vi "Autonomous.vi"   [LabVIEW 2019]
doc: "This VI starts when autonomous period begins, and will automatically be terminated when it ends. You can carry out timed or sensor driven operations directly to I/O or to subsystems without needing to return to the caller."
uses:
  <vilib>/Rock Robotics/WPI/Utilities/WPI_GetSetVariantRefNum.vi
  <vilib>/Rock Robotics/Network Tables/NT Read String.vi
types:
  T1 = typedef "WPI_JoystickDevRef.ctl" = cluster{"Device":T2}
  T2 = typedef "WPI_JoystickDeviceEnum.ctl" = enum16{"USB 0", "USB 1", "USB 2", "USB 3", "USB 4", "USB 5"}
  T3 = typedef "Command Status Info.ctl" = cluster{"Name":string, "Status":T4, "notifier out":T5}
  T4 = typedef "Completion Status.ctl" = enum16{"Successful", "Aborted", "Incomplete"}
  T5 = typedef "Completion Notifier.ctl" = refnum<notifier>
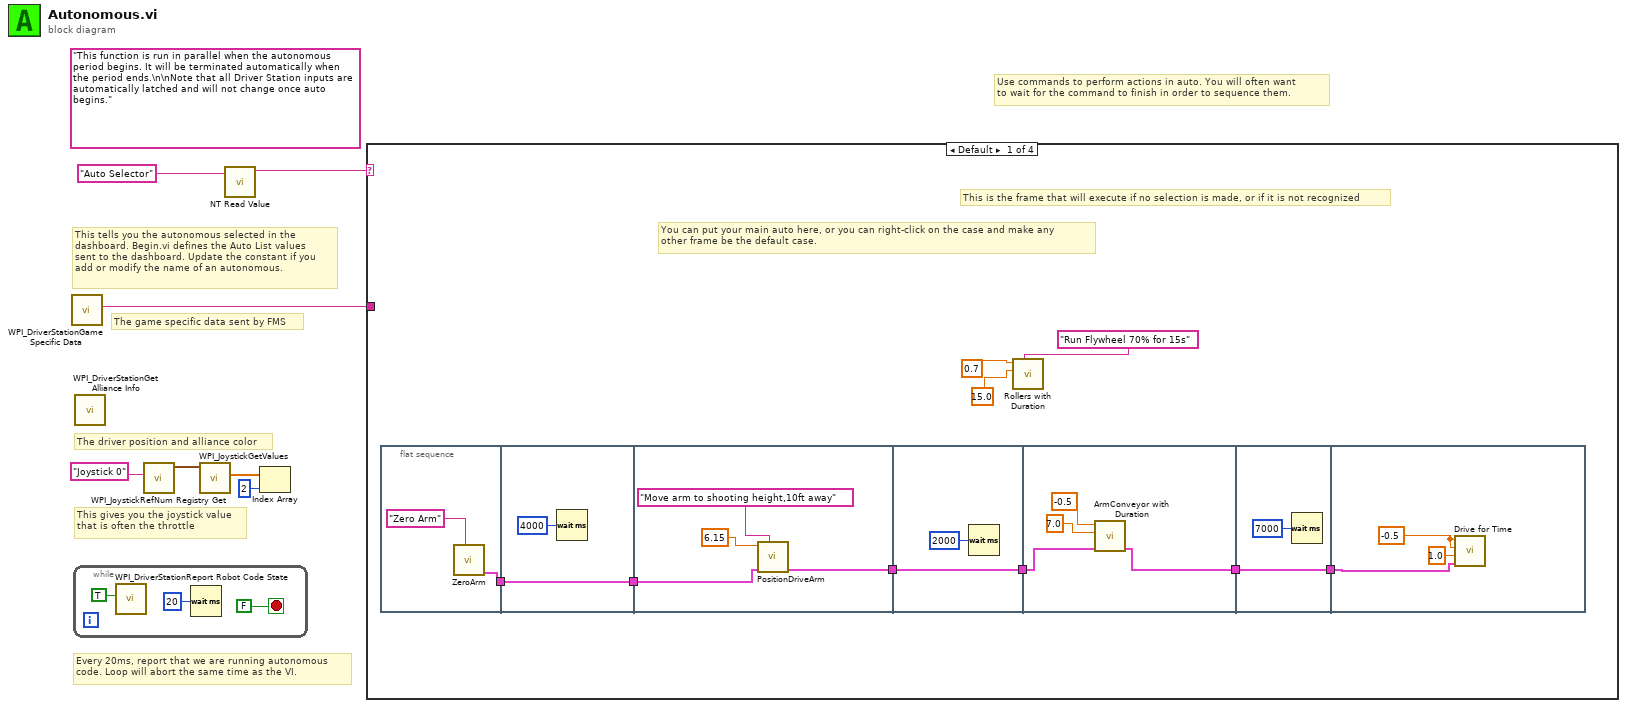
[diagram p0: block diagram]
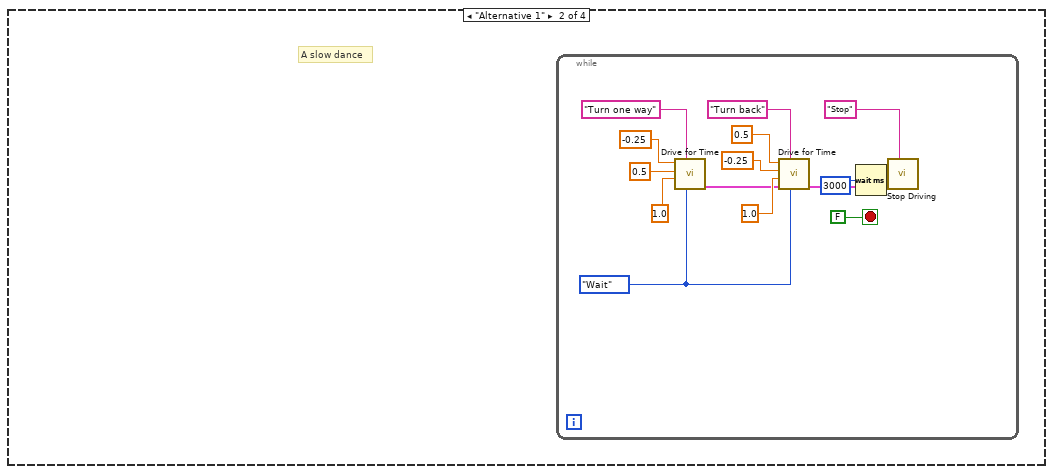
[diagram p2: hidden frame]
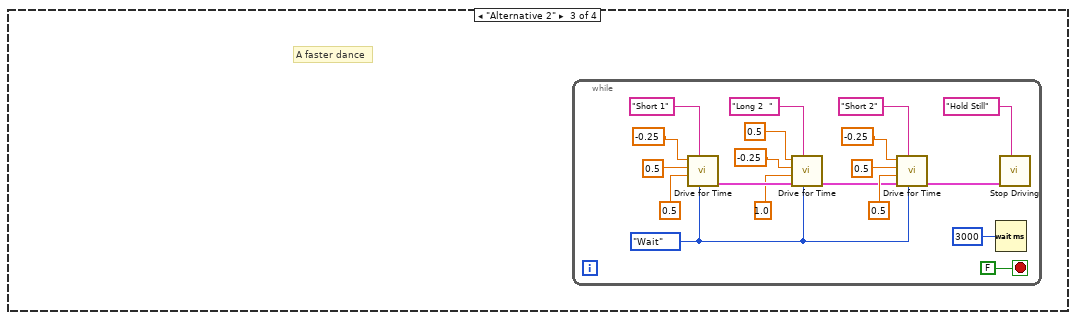
[diagram p3: hidden frame]
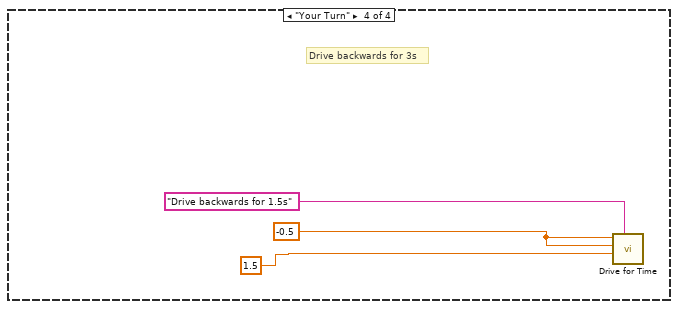
[diagram p4: hidden frame]
diagram:
  (unwired) "This function is run in parallel when the autonomous period begins. It will be terminated automatically when the period ends.\n\nNote that all Driver Station inputs are automatically latched and will not change once auto begins."
  # "The game specific data sent by FMS"
  # "This tells you the autonomous selected in the \ndashboard. Begin.vi defines the Auto List values\nsent to the dashboard. Update the constant if you\nadd or modify the name of an autonomous."
  # "Every 20ms, report that we are running autonomous\ncode. Loop will abort the same time as the VI."
  # "This gives you the joystick value\nthat is often the throttle"
  # "Use commands to perform actions in auto. You will often want\nto wait for the command to finish in order to sequence them."
  # "The driver position and alliance color"
  n1 = call <vilib>:"WPI_DriverStationGame Specific Data.vi"() -> ("Game Specific Data"=w1:string)  [unwired: 11 in]
  n2 = while {
    stop <- FALSE stop-if-true
    n3 = call <vilib>:"WPI_DriverStationReport Robot Code State.vi"("Autonomous"=TRUE) -> ()  [unwired: 10 in, 1 out]
    n4 = Wait (ms)(milliseconds to wait=u32 20) -> ()  [unwired: 1 out]
  }
  n5 = call <vilib>:"WPI_DriverStationGet Alliance Info.vi"() -> ()  [unwired: 12 out]
  n6 = call <vilib>:"WPI_JoystickRefNum Registry Get.vi"("refnum name"="Joystick 0") -> ("JoystickDevRef"=w6:T1)  [unwired: 1 in, 9 out]
  n7 = call <vilib>:"WPI_JoystickGetValues.vi"("JoystickDevRef"=w6) -> ("Axes"=w5:dbl[])  [unwired: 6 in, 4 out]
  n8 = call-poly <vilib>:"NT Read Value.vi"("Name"="Auto Selector") -> ("String"=w2:string)  [unwired: 9 in, 1 out]
  n9 = Index Array(array=w5, index=2) -> ()  [unwired: 1 out]
  n10 = case shown="Default" w2 {
    tunnel: w1 -> [_ _ _ _]
    frame Default {
      # "You can put your main auto here, or you can right-click on the case and make any\nother frame be the default case."
      # "This is the frame that will execute if no selection is made, or if it is not recognized"
      n11 = flat-sequence {
        tunnel: [w20] -> w16
        tunnel: w16 -> [w23]
        tunnel: [w23] -> w15
        tunnel: w15 -> [w24]
        tunnel: [w25] -> w14
        tunnel: w14 -> [w29]
        tunnel: [w29] -> w13
        tunnel: w13 -> [w33]
        tunnel: [w30] -> w12
        tunnel: w12 -> [w35]
        tunnel: [w35] -> w11
        tunnel: w11 -> [w36]
        frame #0 {
          n12 = call "ZeroArm.vi"("Description"="Zero Arm") -> ("Command Info"=w20:T3)  [unwired: 10 in]
        }
        frame #1 {
          n13 = Wait (ms)(milliseconds to wait=u32 4000) -> ()  [unwired: 1 out]
        }
        frame #2 {
          n14 = call "PositionDriveArm.vi"("Description"="Move arm to shooting height,10ft away", "Command Info In"=w24, "Position"=6.15) -> ("Command Info Out"=w25:T3)  [unwired: 8 in]
        }
        frame #3 {
          n15 = Wait (ms)(milliseconds to wait=u32 2000) -> ()  [unwired: 1 out]
        }
        frame #4 {
          n16 = call "ArmConveyor with Duration.vi"("Command Info In"=w33, "Duration (s)"=7.0, "Setpoint"=-0.5) -> ("Command Info Out"=w30:T3)  [unwired: 8 in]
        }
        frame #5 {
          n17 = Wait (ms)(milliseconds to wait=u32 7000) -> ()  [unwired: 1 out]
        }
        frame #6 {
          w37 = -0.5 ("Left Speed")
          n18 = call "Drive for Time.vi"("Command Info In"=w36, "Seconds"=1.0, "Right Speed"=w37, "Left Speed"=w37) -> ()  [unwired: 7 in, 1 out]
        }
      }
      n19 = call "Rollers with Duration.vi"("Description"="Run Flywheel 70% for 15s", "Duration (s)"=15.0, "Setpoint"=0.7) -> ()  [unwired: 8 in, 1 out]
    }
    frame "Alternative 1" {
      # "A slow dance"
      n20 = while {
        stop <- FALSE stop-if-true
        w46 = enum16{"Start", "Wait"}."Wait" ("Synchronication")
        n21 = call "Drive for Time.vi"("Synchronization"=w46, "Description"="Turn one way", "Seconds"=1.0 ("Delay (s)"), "Right Speed"=0.5 ("X axis value"), "Left Speed"=-0.25 ("X axis value")) -> ("Command Info Out"=w40:T3)  [unwired: 6 in]
        n22 = call "Drive for Time.vi"("Synchronization"=w46, "Description"="Turn back", "Command Info In"=w40, "Seconds"=1.0 ("Delay (s)"), "Right Speed"=-0.25 ("X axis value"), "Left Speed"=0.5 ("X axis value")) -> ("Command Info Out"=w47:T3)  [unwired: 5 in]
        n23 = Wait (ms)(milliseconds to wait=u32 3000 ("millisecond timer value")) -> ()  [unwired: 1 out]
        n24 = call "Stop Driving.vi"("Description"="Stop", "Command Info In"=w47) -> ()  [unwired: 9 in, 1 out]
      }
    }
    frame "Alternative 2" {
      # "A faster dance"
      n25 = while {
        stop <- FALSE stop-if-true
        w53 = enum16{"Start", "Wait"}."Wait" ("Synchronication")
        n26 = call "Drive for Time.vi"("Synchronization"=w53, "Description"="Short 1", "Seconds"=0.5 ("Delay (s)"), "Right Speed"=0.5 ("X axis value"), "Left Speed"=-0.25 ("X axis value")) -> ("Command Info Out"=w71:T3)  [unwired: 6 in]
        n27 = call "Drive for Time.vi"("Synchronization"=w53, "Description"="Long 2  ", "Command Info In"=w71, "Seconds"=1.0 ("Delay (s)"), "Right Speed"=-0.25 ("X axis value"), "Left Speed"=0.5 ("X axis value")) -> ("Command Info Out"=w55:T3)  [unwired: 5 in]
        n28 = call "Drive for Time.vi"("Synchronization"=w53, "Description"="Short 2", "Command Info In"=w55, "Seconds"=0.5 ("Delay (s)"), "Right Speed"=0.5 ("X axis value"), "Left Speed"=-0.25 ("X axis value")) -> ("Command Info Out"=w54:T3)  [unwired: 5 in]
        n29 = Wait (ms)(milliseconds to wait=u32 3000 ("millisecond timer value")) -> ()  [unwired: 1 out]
        n30 = call "Stop Driving.vi"("Description"="Hold Still", "Command Info In"=w54) -> ()  [unwired: 9 in, 1 out]
      }
    }
    frame "Your Turn" {
      w72 = -0.5 ("Left Speed")
      # "Drive backwards for 3s"
      n31 = call "Drive for Time.vi"("Description"="Drive backwards for 1.5s", "Seconds"=1.5 ("Right Speed"), "Right Speed"=w72, "Left Speed"=w72) -> ()  [unwired: 7 in, 1 out]
    }
  }
